vi "SeCrTs-RD signal names extracter.vi"(11 "input cluster":T1) -> (1 "Di names":string[](array[string]), 3 "analog names":T2)   [LabVIEW 2022 SP3]
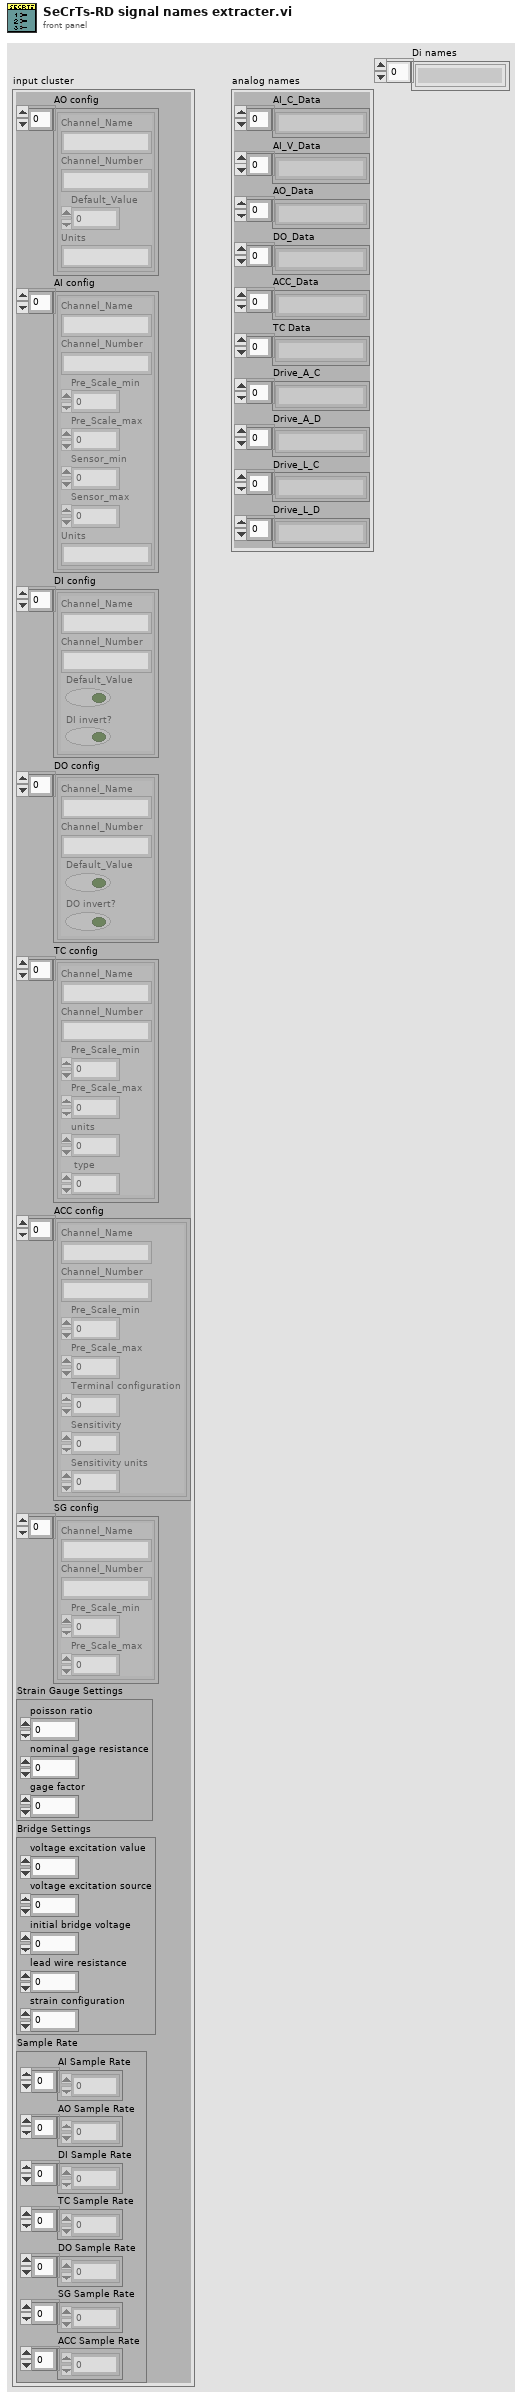
[diagram p1: front panel]
types:
  T1 = cluster{"AO config":cluster{"Channel_Name":string, "Channel_Number":string, "Default_Value":dbl, "Units":string}[], "AI config":cluster{"Channel_Name":string, "Channel_Number":string, "Pre_Scale_min":dbl, "Pre_Scale_max":dbl, "Sensor_min":dbl, "Sensor_max":dbl, "Units":string}[], "DI config":cluster{"Channel_Name":string, "Channel_Number":string, "Default_Value":bool, "DI invert?":bool}[], "DO config":cluster{"Channel_Name":string, "Channel_Number":string, "Default_Value":bool, "DO invert?":bool}[], "TC config":cluster{"Channel_Name":string, "Channel_Number":string, "Pre_Scale_min":dbl, "Pre_Scale_max":dbl, "units":i32, " type":i32}[], "ACC config":cluster{"Channel_Name":string, "Channel_Number":string, "Pre_Scale_min":dbl, "Pre_Scale_max":dbl, "Terminal configuration":i32, "Sensitivity":dbl, "Sensitivity units":i32}[], "SG config":cluster{"Channel_Name":string, "Channel_Number":string, "Pre_Scale_min":dbl, "Pre_Scale_max":dbl}[], "Strain Gauge Settings":cluster{"poisson ratio":dbl, "nominal gage resistance":dbl, "gage factor":dbl}, "Bridge Settings":cluster{"voltage excitation value":dbl, "voltage excitation source":i32, "initial bridge voltage":dbl, "lead wire resistance":dbl, "strain configuration":i32}, "Sample Rate":cluster{"AI Sample Rate":dbl[], "AO Sample Rate":dbl[], "DI Sample Rate":dbl[], "TC Sample Rate":dbl[], "DO Sample Rate":dbl[], "SG Sample Rate":dbl[], "ACC Sample Rate":dbl[]}}
  T2 = cluster{"AI_C_Data":string[], "AI_V_Data":string[], "AO_Data":string[], "DO_Data":string[], "ACC_Data":string[], "TC Data":string[], "Drive_A_C":string[], "Drive_A_D":string[], "Drive_L_C":string[], "Drive_L_D":string[]}
  T3 = cluster{"Channel_Name":string, "Channel_Number":string, "Default_Value":dbl, "Units":string}[]
  T4 = cluster{"Channel_Name":string, "Channel_Number":string, "Pre_Scale_min":dbl, "Pre_Scale_max":dbl, "Sensor_min":dbl, "Sensor_max":dbl, "Units":string}[]
  T5 = cluster{"Channel_Name":string, "Channel_Number":string, "Default_Value":bool, "DI invert?":bool}[]
  T6 = cluster{"Channel_Name":string, "Channel_Number":string, "Default_Value":bool, "DO invert?":bool}[]
  T7 = cluster{"Channel_Name":string, "Channel_Number":string, "Pre_Scale_min":dbl, "Pre_Scale_max":dbl, "units":i32, " type":i32}[]
  T8 = cluster{"Channel_Name":string, "Channel_Number":string, "Pre_Scale_min":dbl, "Pre_Scale_max":dbl, "Terminal configuration":i32, "Sensitivity":dbl, "Sensitivity units":i32}[]
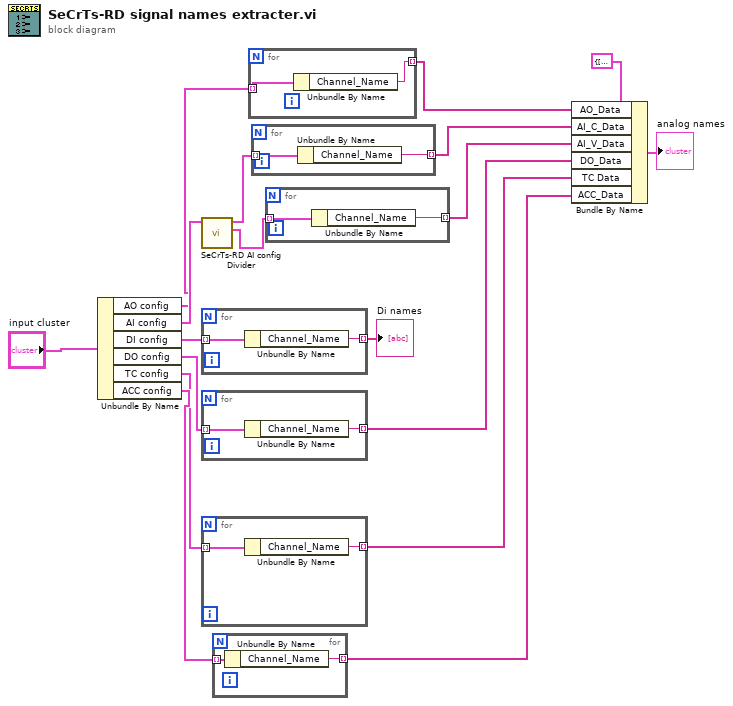
[diagram p0: block diagram]
diagram:
  n1 = Unbundle By Name("input cluster") -> ("AO config"=w2:T3, "AI config"=w9:T4, "DI config"=w3:T5, "DO config"=w4:T6, "TC config"=w5:T7, "ACC config"=w6:T8)
  n2 = call "SeCrTs-RD AI config Divider.vi"("AI config"=w9) -> ("AI V"=w11:T4, "AI C"=w10:T4)  [unwired: 9 in]
  n3 = for {
    tunnel: [w20] -> w1 mode=indexing
    tunnel: w3 -> [w19] mode=indexing
    n4 = Unbundle By Name(w19) -> ("Channel_Name"=w20:string)
  }
  "Di names" <- w1
  n5 = for {
    tunnel: w4 -> [w21] mode=indexing
    tunnel: [w22] -> w14 mode=indexing
    n6 = Unbundle By Name(w21) -> ("Channel_Name"=w22:string)
  }
  n7 = for {
    tunnel: [w24] -> w15 mode=indexing
    tunnel: w5 -> [w23] mode=indexing
    n8 = Unbundle By Name(w23) -> ("Channel_Name"=w24:string)
  }
  n9 = for {
    tunnel: w6 -> [w26] mode=indexing
    tunnel: [w25] -> w16 mode=indexing
    n10 = Unbundle By Name(w26) -> ("Channel_Name"=w25:string)
  }
  n11 = for {
    tunnel: w2 -> [w28] mode=indexing
    tunnel: [w27] -> w7 mode=indexing
    n12 = Unbundle By Name(w28) -> ("Channel_Name"=w27:string)
  }
  n13 = for {
    tunnel: w10 -> [w30] mode=indexing
    tunnel: [w29] -> w12 mode=indexing
    n14 = Unbundle By Name(w30) -> ("Channel_Name"=w29:string)
  }
  n15 = for {
    tunnel: w11 -> [w32] mode=indexing
    tunnel: [w31] -> w13 mode=indexing
    n16 = Unbundle By Name(w32) -> ("Channel_Name"=w31:string)
  }
  n17 = Bundle By Name(cluster=T2 {"AI_C_Data"=[], "AI_V_Data"=[], "AO_Data"=[], "DO_Data"=[], "ACC_Data"=[], "TC Data"=[], "Drive_A_C"=[], "Drive_A_D"=[], "Drive_L_C"=[], "Drive_L_D"=[]} ("Channel names"), "AO_Data"=w7, "AI_C_Data"=w12, "AI_V_Data"=w13, "DO_Data"=w14, "TC Data"=w15, "ACC_Data"=w16) -> (→"analog names":T2)
